vi "Save_cuenta.vi"(8 "error in (no error)":errorcluster, 10 "Cuenta":bool[](array[boolean]), 11 "Logging_Contador_Actor_TDMS in":refnum<class "Logging_Contador_Actor_TDMS.lvclass">) -> (0 "error out":errorcluster, 3 "Logging_Contador_Actor out":refnum<class "Logging_Contador_Actor.lvclass">)   [LabVIEW 2019, in "Logging_Contador_Actor_TDMS.lvlib" / "Logging_Contador_Actor_TDMS.lvclass"]
uses:
  Logging_Contador_Actor_TDMS.lvclass
  C:/Users/Luis/Documents/Ingenieria/Git_versiones/Actor-framework-CML-con-opciones-de-adquisici-n-main/Logging_Contador_Actor/Logging_Contador_Actor/Logging_Contador_Actor.lvclass
  Logging_Contador_Actor/Logging_Contador_Actor/Logging_Contador_Actor.lvclass
  Logging_Contador_Actor/Logging_Contador_Actor/Logging_Contador_Actor.lvclass/Logging_Contador_Actor.ctl
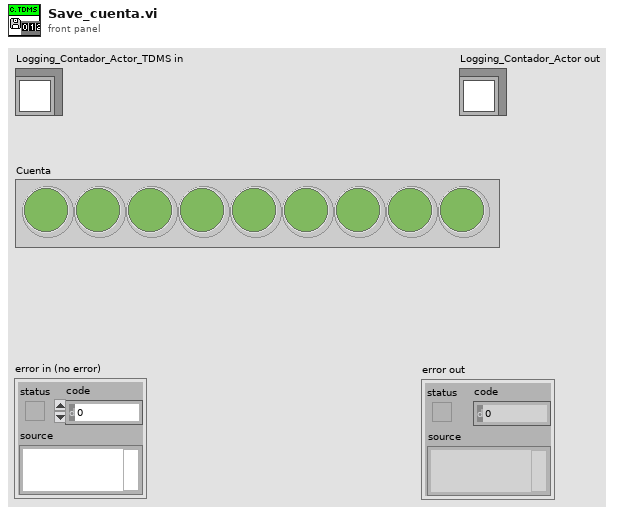
[diagram p1: front panel]
types:
  T1 = enum16{"open", "open or create", "create or replace", "create", "open (read-only)"}
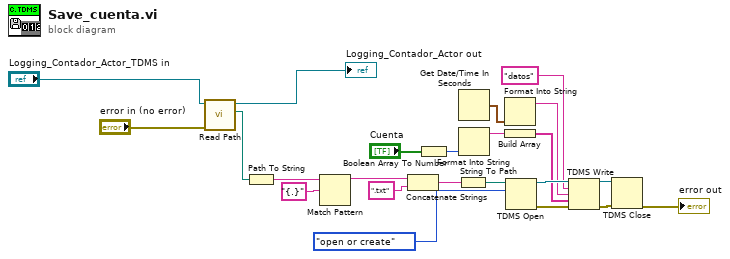
[diagram p0: block diagram]
diagram:
  n1 = call "Read Path.vi"("error in (no error)"="error in (no error)", "Logging_Contador_Actor in"="Logging_Contador_Actor_TDMS in") -> ("Path"=w16:path, "Logging_Contador_Actor out"=→"Logging_Contador_Actor out":refnum<class "Logging_Contador_Actor_TDMS.lvclass">)  [unwired: 7 in, 1 out]
  n2 = Path To String(path=w16) -> (string=w21:string)
  n3 = Match Pattern(string=w21, regular expression="{.}") -> (before substring=w19:string)  [unwired: 1 in, 3 out]
  n4 = Concatenate Strings(w19, ".txt" ("string")) -> (w17:string)
  n5 = Boolean Array To Number(Boolean array="Cuenta") -> (number=w7:u32)
  n6 = String To Path(string=w17) -> (path=w13:path)
  n7 = Get Date/Time In Seconds() -> (seconds since 1Jan1904=w8:timestamp)
  n8 = Format Into String(w7) -> (resulting string=w6:string)  [unwired: 3 in, 1 out]
  n9 = Format Into String(w8) -> (resulting string=w3:string)  [unwired: 3 in, 1 out]
  n10 = Build Array(w6) -> (w5:string[])
  n11 = TDMS Open(10:T1."open or create" ("operation (0:open)"), 11:w13) -> (0:w9:errorcluster, 3:w10:refnum<k34>)  [unwired: 5 in]
  n12 = TDMS Write(0:w10, 5:"datos" ("group name in (Untitled)"), 7:w3, 9:w5, 11:w9) -> (4:w11:refnum<k34>, 15:w12:errorcluster)  [unwired: 1 in, 2 out]
  n13 = TDMS Close(8:w12, 11:w11) -> (0:→"error out":errorcluster)  [unwired: 1 out]
